vi "ReversedEngineering_GetClassPathFromNode.vi"(0 "reference":refnum<class "AbstractNode.lvclass">, 5 "error IO":errorcluster) -> (15 "Path":path, 19 "error out":errorcluster)   [LabVIEW 2014]
uses:
  <resource>/Framework/Providers/Open_GDS/UML/AbstractNode_class/AbstractNode.lvclass
  <resource>/Framework/Providers/Open_GDS/UML/ClassNode_class/ExternalSetTypes.ctl
  <resource>/Framework/Providers/Open_GDS/UML/ClassNode_class/ClassNode.lvclass
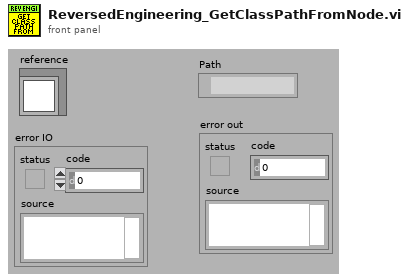
[diagram p1: front panel]
types:
  T1 = typedef "ClassNode.lvclass/ExternalSetTypes.ctl" = enum16{"Name", "Attributes", "Methods", "Position", "ShowMethods", "ShowAttributes", "ClassPath"}
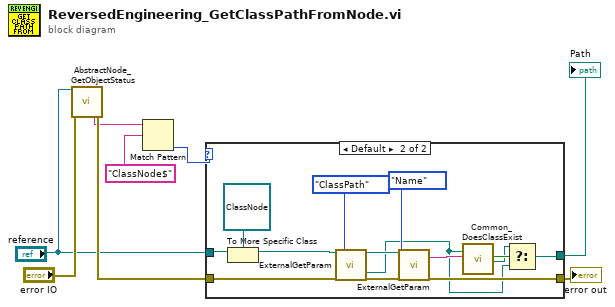
[diagram p0: block diagram]
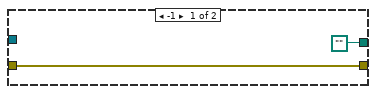
[diagram p2: hidden frame]
diagram:
  n1 = call <resource>:"AbstractNode_GetObjectStatus.vi"("reference in"="reference", "error in (no error)"="error IO") -> ("Class name"=w3:string, "error out"=w6:errorcluster)  [unwired: 16 out]
  n2 = Match Pattern(string=w3, regular expression="ClassNode$") -> (offset past match=w8:i32)  [unwired: 4 out]
  n3 = case shown="Default" w8 {
    tunnel: "reference" -> [_ w13]
    tunnel: w6 -> [w10 w14]
    tunnel: [w10 w19] -> w1
    tunnel: [path "" w15] -> w2
    frame -1 {
    }
    frame Default {
      n4 = To More Specific Class(target class=refnum<class "ClassNode.lvclass"> refnum ("reference"), reference=w13) -> (specific class reference=w11:refnum<class "ClassNode.lvclass">)  [unwired: 1 in, 1 out]
      n5 = call <resource>:"ExternalGetParam.vi"("reference"=w11, "setParameter"=ExternalSetTypes."ClassPath", "error in (no error)"=w14) -> ("reference out"=w23:refnum<class "ClassNode.lvclass">, "Path"=w17:path, "error out"=w22:errorcluster)  [unwired: 14 out]
      n6 = call <resource>:"ExternalGetParam.vi"("reference"=w23, "setParameter"=ExternalSetTypes."Name", "error in (no error)"=w22) -> ("string"=w20:string, "error out"=w19:errorcluster)  [unwired: 15 out]
      n7 = call <resource>:"Common_DoesClassExist.vi"("ClassPath"=w17, "ClassName"=w20) -> ("llb-class"=w18:bool, "llb/LvCLass-Path"=w16:path)  [unwired: 16 out]
      n8 = Select(t=w16, s=w18, f=w17) -> (s? t:f=w15:path)
    }
  }
  "Path" <- w2
  "error out" <- w1
